vi "AlliGator Phasor Plot Mouse Move Flag.vi"(2 "Flag (in)":bool, 4 "Read/Write":T1) -> (7 "Flag (out)":bool)   [LabVIEW 2021, in "AlliGator Phasor Plot.lvlib"]
doc: "Raise the flag when calling the action.\nLower it when done."
uses:
  Utilities/Read-Write.ctl
  AlliGator Phasor Plot.lvlib
  Utilities/Utilities.lvlib
panel:
  # "see the AlliGator License on the block diagram (Ctrl+E or Window:Show Block Diagram)"
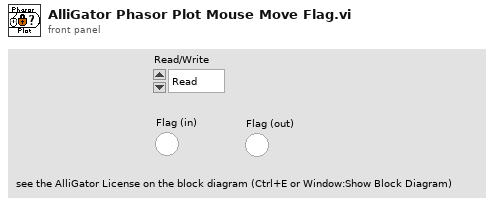
[diagram p1: front panel]
types:
  T1 = typedef "Utilities.lvlib/Read-Write.ctl" = enum16{"Read", "Write"}
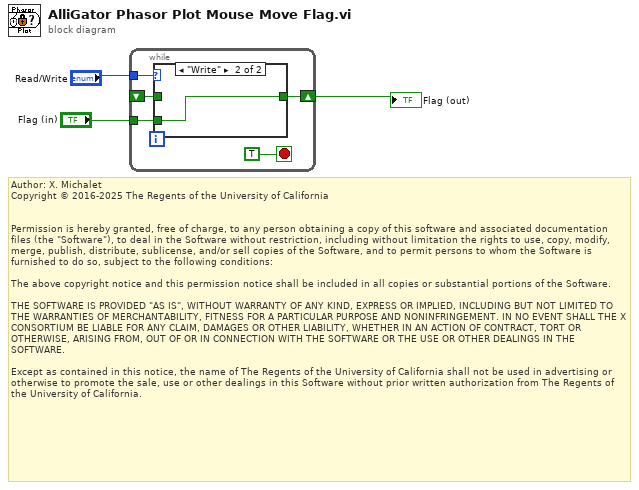
[diagram p0: block diagram]
diagram:
  # "Author: X. Michalet\nCopyright © 2016-2025 The Regents of the University of California\n \n\nPermission is hereby granted, free of charge, to any person obtaining a copy of this software and associated documentation files (the \"Software\"), to deal in the Software without restriction, including without limitation the rights to use, copy, modify, merge, publish, distribute, sublicense, and/or sell copies of the Software, and to permit persons to whom the Software is furnished to do so, subject to the following conditions:\n\nThe above copyright notice and this permission notice shall be included in all copies or substantial portions of the Software.\n\nTHE SOFTWARE IS PROVIDED \"AS IS\", WITHOUT WARRANTY OF ANY KIND, EXPRESS OR IMPLIED, INCLUDING BUT NOT LIMITED TO THE WARRANTIES OF MERCHANTABILITY, FITNESS FOR A PARTICULAR PURPOSE AND NONINFRINGEMENT. IN NO EVENT SHALL THE X CONSORTIUM BE LIABLE FOR ANY CLAIM, DAMAGES OR OTHER LIABILITY, WHETHER IN AN ACTION OF CONTRACT, TORT OR OTHERWISE, ARISING FROM, OUT OF OR IN CONNECTION WITH THE SOFTWARE OR THE USE OR OTHER DEALINGS IN THE SOFTWARE.\n\nExcept as contained in this notice, the name of The Regents of the University of California shall not be used in advertising or otherwise to promote the sale, use or other dealings in this Software without prior written authorization from The Regents of the University of California."
  n1 = while {
    tunnel: "Read/Write" -> [w7]
    shift-right: [w5] -> w1
    shift-left: _ -> [w6]
    tunnel: "Flag (in)" -> [w4]
    stop <- TRUE stop-if-true
    n2 = case shown="\"Write\"" w7 {
      tunnel: w6 -> [w9 _]
      tunnel: [w9 w10] -> w5
      tunnel: w4 -> [_ w10]
      frame "Read", Default {
      }
      frame "Write" {
      }
    }
  }
  "Flag (out)" <- w1
